vi "dev_make-gaussian-2d.vi"(9 "StdDev":dbl[](array[numeric]), 10 "Mean":dbl[](array[numeric]), 11 "in":dbl[](array[numeric]) format="%#_13g") -> (3 "out":dbl)   [LabVIEW 2024]
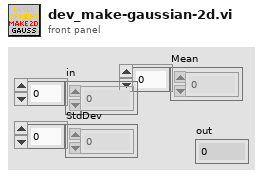
[diagram p1: front panel]
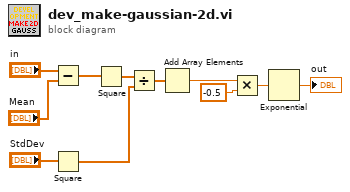
[diagram p0: block diagram]
diagram:
  n1 = Subtract(x="in", y="Mean") -> (x-y=w5:dbl[])
  n2 = Square(x="StdDev") -> (x^2=w7:dbl[])
  n3 = Square(x=w5) -> (x^2=w6:dbl[])
  n4 = Divide(x=w6, y=w7) -> (x/y=w8:dbl[])
  n5 = Add Array Elements(numeric array=w8) -> (sum=w1:dbl)
  n6 = Multiply(x=w1, y=-0.5) -> (x*y=w10:dbl)
  n7 = Exponential(1:w10) -> (0:→"out":dbl)
